vi "ColorTemp.vi"(0 "DeviceNo":u32, 1 "Mode":u16(ring) items=["Get&Set", "Get", "Set"], 5 "ChildNo":u32, 11 "Error_In":T1, 12 "SetColor":cluster{"Mode":u32, "R":u32, "G":u32, "B":u32}) -> (3 "ColorTempList":cluster{string, i32}[](array[cluster]), 4 "Error?":bool, 6 "Base":u32, 8 "Type":i8, 10 "Max":u32, 14 "GetColor":cluster{"Mode":u32, "R":u32, "G":u32, "B":u32}, 15 "Error_Out":T1)   [LabVIEW 2015]
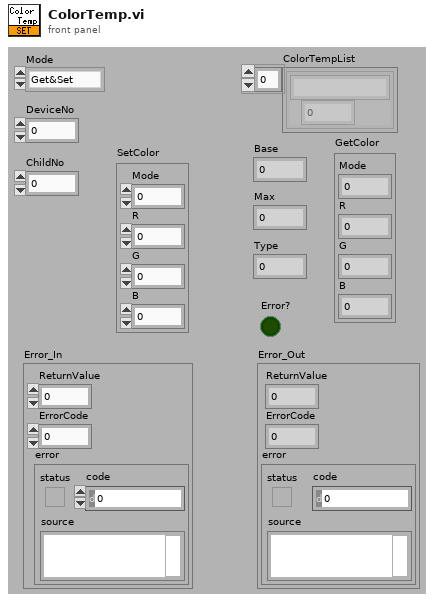
[diagram p1: front panel]
types:
  T1 = cluster{"ReturnValue":u32, "ErrorCode":u32, "error ":errorcluster}
  T2 = cluster{"pMode":u32, "pR":u32, "pG":u32, "pB":u32}
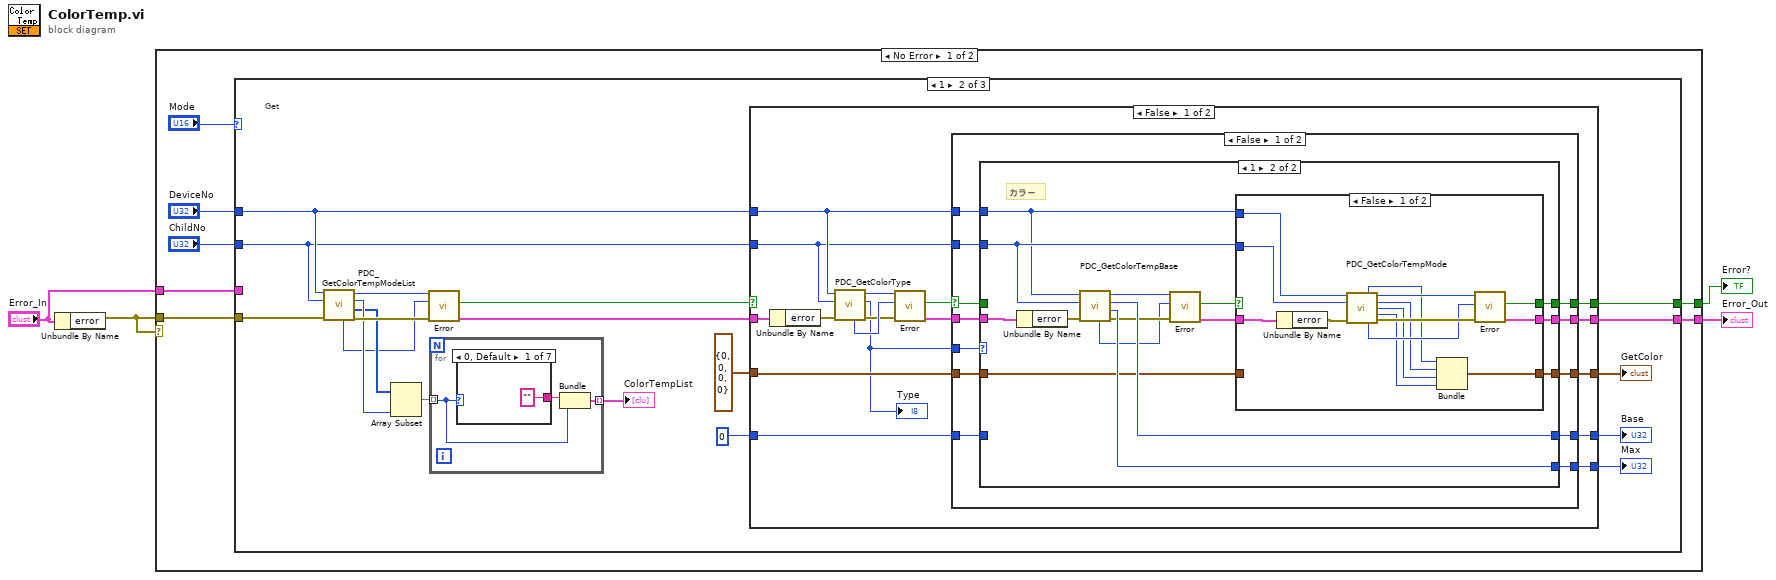
[diagram p0: block diagram]
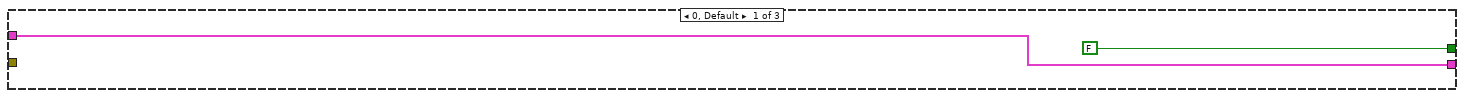
[diagram p2: hidden frame]
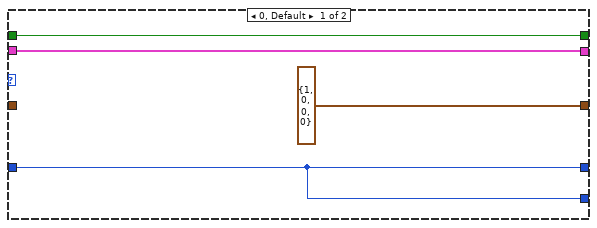
[diagram p3: hidden frame]
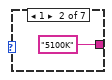
[diagram p7: hidden frame]
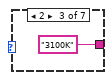
[diagram p8: hidden frame]
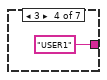
[diagram p9: hidden frame]
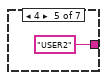
[diagram p10: hidden frame]
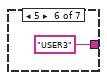
[diagram p11: hidden frame]
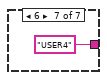
[diagram p12: hidden frame]
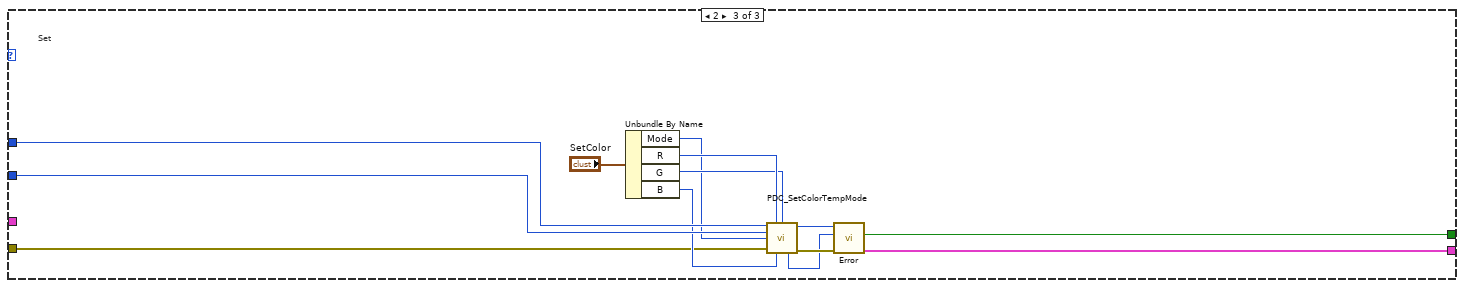
[diagram p13: hidden frame]
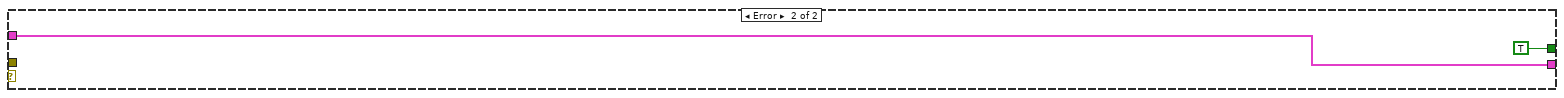
[diagram p14: hidden frame]
diagram:
  n1 = Unbundle By Name("Error_In") -> ("error"=w1:errorcluster)
  n2 = case shown="No Error" w1 {
    tunnel: [w8 TRUE ("Error?")] -> w4
    tunnel: [w7 w130] -> w3
    tunnel: w1 -> [w6 _]
    tunnel: "Error_In" -> [w5 w130]
    frame No Error {
      n3 = case shown="1" "Mode" {
        tunnel: "DeviceNo" -> [_ w23 w123]
        tunnel: "ChildNo" -> [_ w22 w122]
        tunnel: [FALSE ("Error?") w21 w124] -> w8
        tunnel: [w12 w20 w125] -> w7
        tunnel: w6 -> [_ w14 w116]
        tunnel: w5 -> [w12 _ _]
        frame 0, Default {
        }
        frame 1 {
          # "Get"
          n4 = call "PDC_GetColorTempModeList.vi"("error in (no error)"=w14, "ChildNo"=w22, "DeviceNo"=w23) -> ("error out"=w28:errorcluster, "List"=w26:u32[], "Size"=w27:u32, "ReturnValue"=w29:u32, "ErrorCode"=w25:u32)  [unwired: 4 out]
          n5 = Array Subset(array=w26, length=w27) -> (w31:u32[])  [unwired: 1 in]
          n6 = call "Error.vi"("error in (no error)"=w28, "ErrorCode"=w25, "ReturnValue"=w29) -> ("Error_Out"=w32:T1, "Error?"=w24:bool)  [unwired: 7 out]
          n7 = for {
            tunnel: w31 -> [w107] mode=indexing
            tunnel: [w106] -> w30 mode=indexing
            n8 = case shown="0, Default" w107 {
              tunnel: ["" "5100K" "3100K" "USER1" "USER2" "USER3" "USER4"] -> w108
              frame 0, Default {
              }
              frame 1 {
              }
              frame 2 {
              }
              frame 3 {
              }
              frame 4 {
              }
              frame 5 {
              }
              frame 6 {
              }
            }
            n9 = Bundle(w108, "pList"=w107) -> (w106:cluster{string, "pList":u32})  [unwired: 1 out]
          }
          "ColorTempList" <- w30
          n10 = case shown="False" w24 {
            selector: w24 -> [_ w104]
            tunnel: w32 -> [w41 w105]
            tunnel: w23 -> [w47 _]
            tunnel: w22 -> [w46 _]
            tunnel: [w49 w104] -> w21
            tunnel: [w48 w105] -> w20
            tunnel: [w38 w103] -> w19
            tunnel: T2 {"pMode"=0, "pR"=0, "pG"=0, "pB"=0} -> [w37 w103]
            tunnel: [w36 w102] -> w17
            tunnel: [w35 w102] -> w16
            tunnel: u32 0 ("pBase") -> [w34 w102]
            frame False {
              n11 = Unbundle By Name(w41) -> ("error"=w39:errorcluster)
              n12 = call "PDC_GetColorType.vi"("error in (no error)"=w39, "ChildNo"=w46, "DeviceNo"=w47) -> ("error out"=w43:errorcluster, "Mode"=w33:i8, "ReturnValue"=w45:u32, "ErrorCode"=w44:u32)  [unwired: 5 out]
              "Type" <- w33
              n13 = call "Error.vi"("error in (no error)"=w43, "ErrorCode"=w44, "ReturnValue"=w45) -> ("Error_Out"=w40:T1, "Error?"=w42:bool)  [unwired: 7 out]
              n14 = case shown="False" w42 {
                selector: w42 -> [w51 w100]
                tunnel: w46 -> [w61 _]
                tunnel: w47 -> [w60 _]
                tunnel: w40 -> [w59 w101]
                tunnel: [w58 w100] -> w49
                tunnel: [w57 w101] -> w48
                tunnel: [w56 w99] -> w38
                tunnel: w37 -> [w53 w99]
                tunnel: [w55 w98] -> w36
                tunnel: [w54 w98] -> w35
                tunnel: w34 -> [w50 w98]
                tunnel: w33 -> [w52 _]
                frame False {
                  n15 = case shown="1" w52 {
                    tunnel: w61 -> [_ w80]
                    tunnel: w60 -> [_ w79]
                    tunnel: w59 -> [w65 w78]
                    tunnel: [w64 w77] -> w58
                    tunnel: [w65 w76] -> w57
                    tunnel: [T2 {"pMode"=1, "pR"=0, "pG"=0, "pB"=0} w75] -> w56
                    tunnel: [w62 w74] -> w55
                    tunnel: [w62 w73] -> w54
                    tunnel: w53 -> [_ w70]
                    tunnel: w51 -> [w64 _]
                    tunnel: w50 -> [w62 _]
                    frame 0, Default {
                    }
                    frame 1 {
                      # "カラー"
                      n16 = Unbundle By Name(w78) -> ("error"=w69:errorcluster)
                      n17 = call "PDC_GetColorTempBase.vi"("error in (no error)"=w69, "ChildNo"=w80, "DeviceNo"=w79) -> ("error out"=w68:errorcluster, "Max"=w73:u32, "Base"=w74:u32, "ReturnValue"=w67:u32, "ErrorCode"=w66:u32)  [unwired: 4 out]
                      n18 = call "Error.vi"("error in (no error)"=w68, "ErrorCode"=w66, "ReturnValue"=w67) -> ("Error_Out"=w72:T1, "Error?"=w71:bool)  [unwired: 7 out]
                      n19 = case shown="False" w71 {
                        selector: w71 -> [_ w96]
                        tunnel: [w83 w97] -> w76
                        tunnel: [w84 w96] -> w77
                        tunnel: w72 -> [w94 w97]
                        tunnel: w79 -> [w93 _]
                        tunnel: w80 -> [w92 _]
                        tunnel: [w81 w95] -> w75
                        tunnel: w70 -> [_ w95]
                        frame False {
                          n20 = Unbundle By Name(w94) -> ("error"=w91:errorcluster)
                          n21 = call "PDC_GetColorTempMode.vi"("DeviceNo"=w93, "ChildNo"=w92, "error in (no error)"=w91) -> ("Mode"=w82:u32, "ReturnValue"=w90:u32, "R"=w87:u32, "G"=w86:u32, "B"=w85:u32, "ErrorCode"=w88:u32, "error out"=w89:errorcluster)  [unwired: 6 out]
                          n22 = Bundle("Mode"=w82, "R"=w87, "G"=w86, "B"=w85) -> (w81:cluster{"Mode":u32, "R":u32, "G":u32, "B":u32})  [unwired: 1 out]
                          n23 = call "Error.vi"("error in (no error)"=w89, "ErrorCode"=w88, "ReturnValue"=w90) -> ("Error_Out"=w83:T1, "Error?"=w84:bool)  [unwired: 7 out]
                        }
                        frame True {
                        }
                      }
                    }
                  }
                }
                frame True {
                }
              }
            }
            frame True {
            }
          }
          "Base" <- w17
          "Max" <- w16
          "GetColor" <- w19
        }
        frame 2 {
          # "Set"
          n24 = Unbundle By Name("SetColor") -> ("Mode"=w117:u32, "R"=w119:u32, "G"=w118:u32, "B"=w120:u32)
          n25 = call "PDC_SetColorTempMode.vi"("DeviceNo"=w123, "R"=w119, "G"=w118, "ChildNo"=w122, "Mode"=w117, "error in (no error)"=w116, "B"=w120) -> ("ReturnValue"=w127:u32, "ErrorCode"=w126:u32, "error out"=w128:errorcluster)  [unwired: 6 out]
          n26 = call "Error.vi"("error in (no error)"=w128, "ErrorCode"=w126, "ReturnValue"=w127) -> ("Error_Out"=w125:T1, "Error?"=w124:bool)  [unwired: 7 out]
        }
      }
    }
    frame Error {
    }
  }
  "Error_Out" <- w3
  "Error?" <- w4
